vi "HSDIO Test Out.vi"() -> ()   [LabVIEW 2010]
uses:
  <vilib>/eio/EIONode/EIONode.xnode
  <vilib>/rvi/eio/nirviEIOImplementation/nirviEIOImplementation.xnode
  <vilib>/rvi/eio/common/nirviEmuClasses.ctl
  <vilib>/rvi/eio/common/nirviEmuTemplateMethod_noerrors.vi
panel:
  in  "Count(mSec)":u32=200
  out "Lidar Cable Check":bool
  in  "stop 2":bool
  in  "stop":bool
  out "Heartbeat":bool
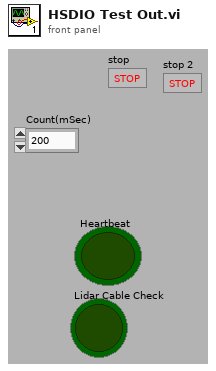
[diagram p1: front panel]
types:
  T1 = typedef "nirviEmuClasses.ctl" = enum16{"IO Read", "IO Write", "Method", "Property Read", "Property Write"}
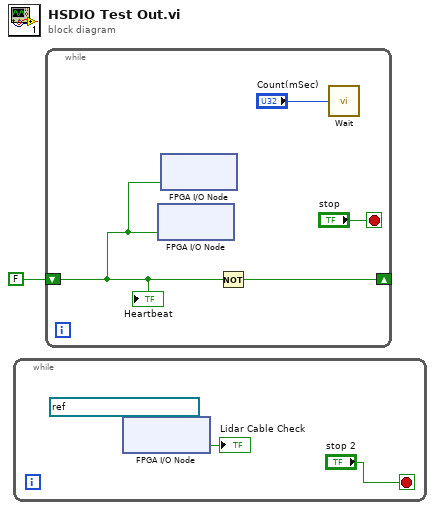
[diagram p0: block diagram]
diagram:
  n1 = while {
    stop <- "stop 2" stop-if-true
    n2 = xnode "FPGA I/O Node"("FPGA I/O In"=refnum<k21> "Lidar Data Cable Check") -> ("I/O Item"=→"Lidar Cable Check":bool)  [unwired: 1 out]
  }
  n3 = while {
    shift-right: [w26] -> _
    shift-left: FALSE -> [w24]
    stop <- "stop" stop-if-true
    n4 = xnode "FPGA I/O Node"("Rx"=w24) -> ()  [unwired: 1 in, 1 out]
    n5 = xnode "FPGA I/O Node"("Tx"=w24) -> ()  [unwired: 1 in, 1 out]
    n6 = Not(x=w24) -> (.not. x?=w26:bool)
    n7 = call "Wait"("Count(mSec)"="Count(mSec)") -> ()  [unwired: 1 out]
    "Heartbeat" <- w24
  }
